vi "ControllerIdentification.vi"() -> ()   [LabVIEW 2013]
panel:
  out "Identification":string
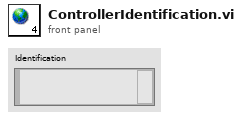
[diagram p1: front panel]
diagram:
